vi "PH_gentec_Powermeter.Standard Connection Handler.vi"(2 "Connection in":T1, 3 "Timeout":bool, 4 "Device Error":errorcluster, 5 "Error":string) -> (0 "No problem":bool, 1 "Connection out":T1)   [LabVIEW 2014, in "PH_gentec_Powermeter.lvlib"]
uses:
  PH_gentec_Powermeter.lvlib
  PH_Powermeter_BaseClass/PH_Powermeter_BaseClass.Connection.ctl
  PH_Powermeter_BaseClass/PH_Powermeter_BaseClass.State.ctl
  PH_Powermeter_BaseClass/PH_Powermeter_BaseClass.lvlib
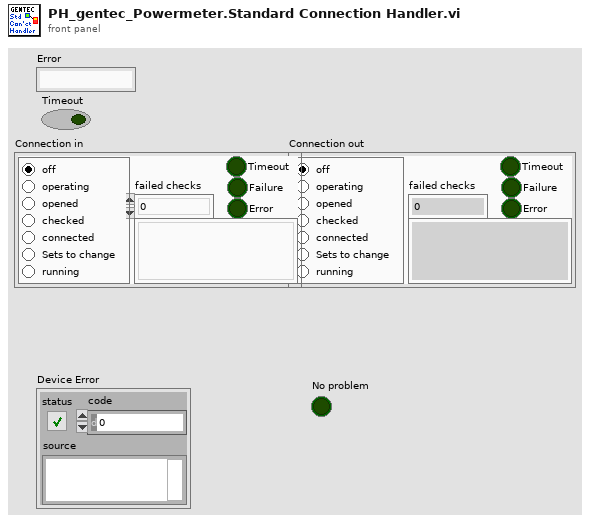
[diagram p1: front panel]
types:
  T1 = typedef "PH_Powermeter_BaseClass.lvlib/PH_Powermeter_BaseClass.Connection.ctl" = cluster{"failed checks":i8, "Timeout":bool, "Data read":string, "Failure":bool, "Error":bool, "State":T2}
  T2 = typedef "PH_Powermeter_BaseClass.lvlib/PH_Powermeter_BaseClass.State.ctl" = enum32{"off", "operating", "opened", "checked", "connected", "Sets to change", "running"}
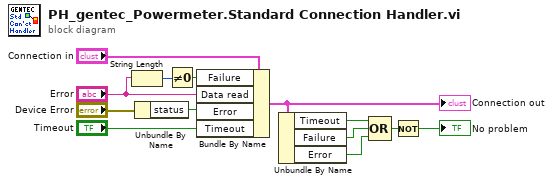
[diagram p0: block diagram]
diagram:
  n1 = String Length(string="Error") -> (length=w12:i32)
  n2 = Unbundle By Name("Device Error") -> ("status"=w9:bool)
  n3 = Not Equal To 0?(x=w12) -> (x != 0?=w13:bool)
  n4 = Bundle By Name(cluster="Connection in", "Failure"=w13, "Data read"="Error", "Error"=w9, "Timeout"="Timeout") -> (w6:T1)
  "Connection out" <- w6
  n5 = Unbundle By Name(w6) -> ("Timeout"=w5:bool, "Failure"=w4:bool, "Error"=w3:bool)
  n6 = Compound Arithmetic op=OR(w5, w4, w3) -> (w2:bool)
  n7 = Not(x=w2) -> (.not. x?=→"No problem":bool)
